vi "GUI.ventana errores.vi"() -> ()   [LabVIEW 2009]
uses:
  Machine State.ctl
panel:
  out "Error Text":string
  in  "Error Code":i32
  out "error out":errorcluster
  in  "error in (no error) 2":errorcluster
  in  "States":T1=enum."Init"
  in  "Array":T1[](array[typedef])
  in  "Which Button?":T2(ring)=enum."Center Button"
  in  "VENTANITA":enum32{"Page 1", "Page 2"}(tab)
  out "Numero error":string
  out "Ultimos LLamadas":string[][](table)
  out "Ultimos Estados":string[][](table)
  # "ERROR EN LABVIEW!!!!"
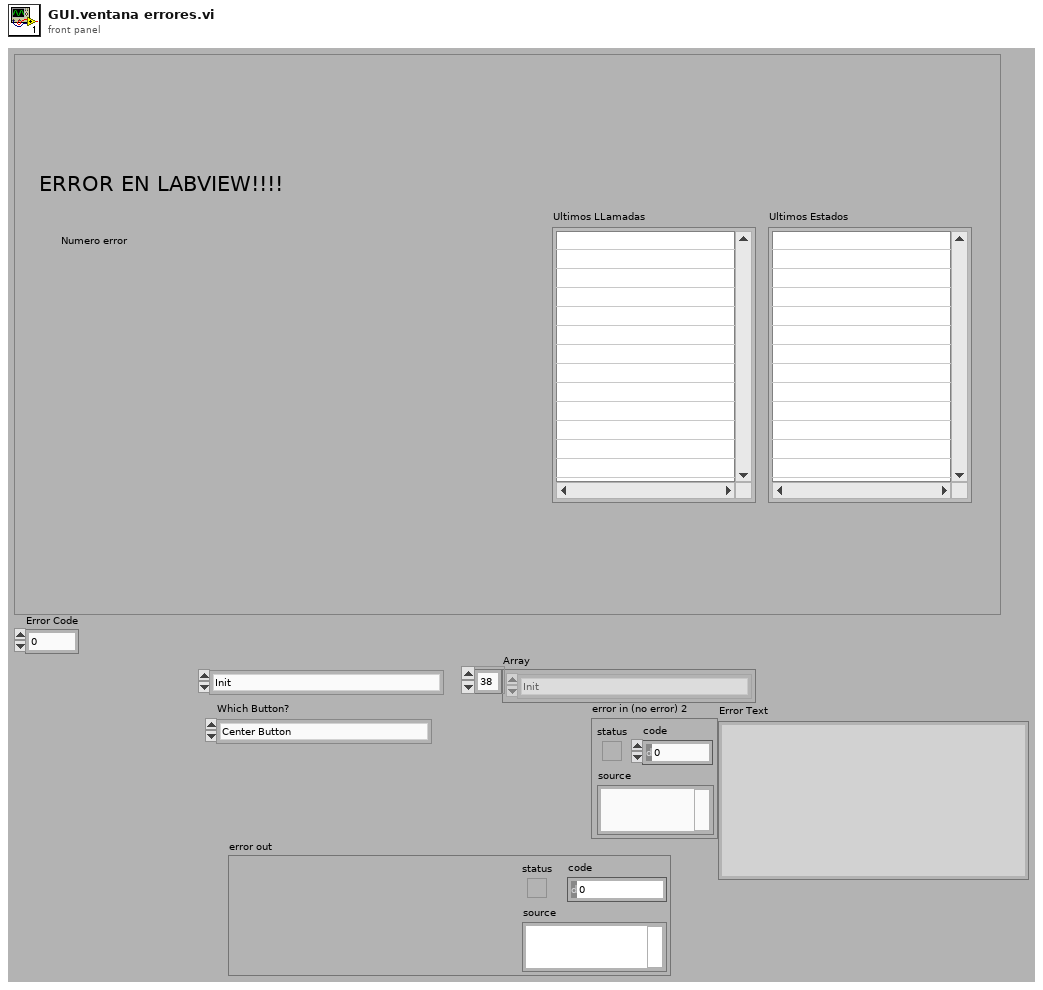
[diagram p1: front panel]
types:
  T1 = typedef "Machine State.ctl" = enum16{"Load temporal config", "Oscilloscope & Pulse Generator Start", "Init", "Config Test", "Start test", "Power Supply", "Osciloscope & Pulse check", "Link FT232", "Seleccion Vasic", "Guardar Valor HW", "Asic Registers", "Board Test. ADC", "Asic Max Min N P", "Adc count", "Asic Rate Scan", "Asic Rate Scan Adders", "Asic Analog Offset", "Asic Digital Offset", "Ft232 Stop", "Oscilloscope & Pulse Generator Stop", "Power Stop", "Loop Vasic", "Stop Test", "Report Partial", "Generate Report", "Check exit", "Exit", "Bye bye Julai", "Error"}
  T2 = enum16{"Left Button", "Center Button", "Right Button", "Window Close"}
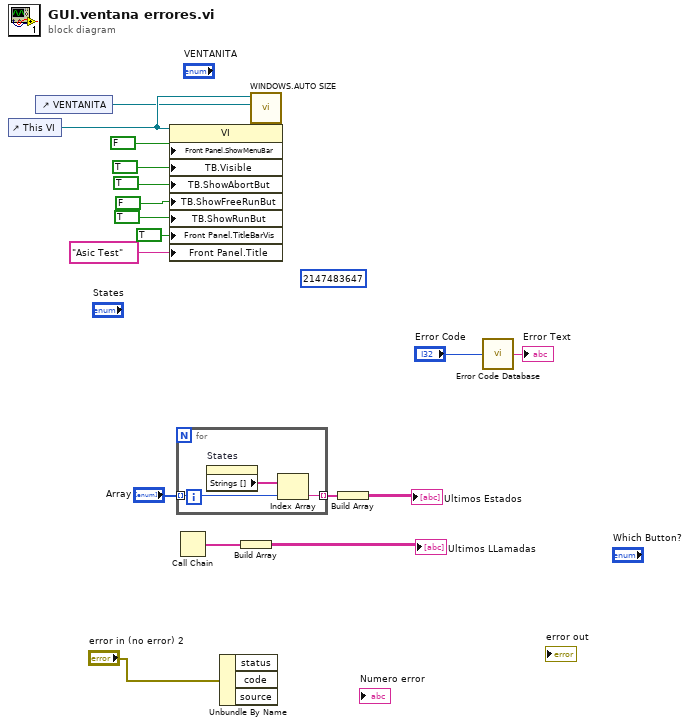
[diagram p0: block diagram]
diagram:
  (unwired) 2147483647
  n1 = control-ref of="This VI"() -> (w15:refnum<vi>)
  n2 = control-ref of="VENTANITA"() -> (w14:refnum<vi>)
  n3 = property class="VI"(reference=w15, "Front Panel.ShowMenuBar"=FALSE ("Front Panel Window:Title Bar Visible"), "TB.Visible"=TRUE ("Front Panel Window:Show Menu Bar"), "TB.ShowAbortBut"=TRUE ("Front Panel Window:Show Menu Bar"), "TB.ShowFreeRunBut"=FALSE ("Front Panel Window:Show Menu Bar"), "TB.ShowRunBut"=TRUE ("Front Panel Window:Show Menu Bar"), "Front Panel.TitleBarVis"=TRUE ("Front Panel Window:Title Bar Visible"), "Front Panel.Title"="Asic Test" ("Front Panel Window:Title")) -> ()  [unwired: 1 in, 2 out]
  n4 = for {
    tunnel: "Array" -> [w19] mode=indexing
    tunnel: [w18] -> w7 mode=indexing
    n5 = property on="States" class="Enum (strict)"() -> ("Strings []"=w20:string[])  [unwired: 2 in, 2 out]
    n6 = Index Array(array=w20, index=w19) -> (element=w18:string)
  }
  n7 = Call Chain() -> (call chain=w5:string[])
  n8 = Unbundle By Name("error in (no error) 2") -> ()  [unwired: 3 out]
  n9 = Build Array(w5) -> (→"Ultimos LLamadas":string[][])
  n10 = call "WINDOWS.AUTO SIZE.vi"("TAB.AutoAjuste"=w14, "This VI"=w15) -> ()  [unwired: 5 in, 1 out]
  n11 = Build Array(w7) -> (→"Ultimos Estados":string[][])
  n12 = call <vilib>:"Error Code Database.vi"("Error Code"="Error Code") -> ("Error Text"=→"Error Text":string)
